vi "pmu_Build Class CFG.vi"(8 "error in (no error)":errorcluster, 11 "CFG input":T1={"PMU ID"=0, "time base"=10000000, "nominal frequency"=enum."60 Hz", "reporting rate"=60, "station name"="", "data format"=15, "phasor channels"=[], "analog channels"=[], "digital channels"=[]} {"digital channels"."digital unit" format="%08x"; "analog channels"."analog unit" format="%08x"; "phasor channels"."phasor unit scaling" max=16777215 format="%06x"; "phasor channels"."phasor unit" items=["Voltage [V]"=0, "Current [A]"=16777216]; "data format" format="%016b"}) -> (0 "error out":errorcluster, 3 "CFG class":T5={"station name"="", "PMU ID"=0, "time base"=10000000, "nominal frequency"=enum."60 Hz", "reporting rate"=60, "phasor number"=0, "analog number"=0, "digital number"=0, "channel names"=[], "phasor units"=[], "analog units"=[], "digital units"=[], "data format"=15, "number of PMUs"=1} {"digital units" format="%.0x"; "analog units" format="%.0x"; "phasor units" format="%.0x"})   [LabVIEW 2013, in "NI_EP_PMU.lvlib"]
uses:
  <vilib>/addons/Electrical Power/PMU/NI_EP_PMU.lvlib
  <vilib>/addons/Electrical Power/PMU/Common/Controls/pmu_CFG Class.ctl
  <vilib>/addons/Electrical Power/PMU/Common/Controls/pmu_CFG Input.ctl
  <vilib>/addons/Electrical Power/PMU/Common/Controls/pmu_Phasor Channel.ctl
  <vilib>/addons/Electrical Power/PMU/Common/Controls/pmu_Analog Channel.ctl
  <vilib>/addons/Electrical Power/PMU/Common/Controls/pmu_Digital Channel.ctl
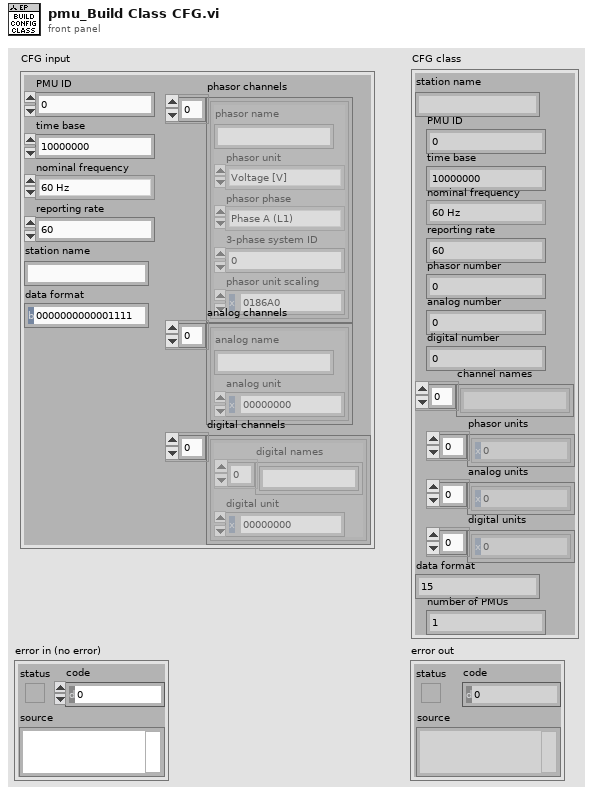
[diagram p1: front panel]
types:
  T1 = typedef "NI_EP_PMU.lvlib/pmu_CFG Input.ctl" = cluster{"PMU ID":u16, "time base":u32, "nominal frequency":enum16{"50 Hz", "60 Hz"}, "reporting rate":i16, "station name":string, "data format":u16, "phasor channels":T2[], "analog channels":T3[], "digital channels":T4[]}
  T2 = typedef "NI_EP_PMU.lvlib/pmu_Phasor Channel.ctl" = cluster{"phasor name":string, "phasor unit":u32, "phasor phase":enum16{"Phase A (L1)", "Phase B (L2)", "Phase C (L3)", "Phase N", "Positive sequence", "Negative sequence", "Zero sequence"}, "3-phase system ID":u8, "phasor unit scaling":u32}
  T3 = typedef "NI_EP_PMU.lvlib/pmu_Analog Channel.ctl" = cluster{"analog name":string, "analog unit":u32}
  T4 = typedef "NI_EP_PMU.lvlib/pmu_Digital Channel.ctl" = cluster{"digital names":string[], "digital unit":u32}
  T5 = typedef "NI_EP_PMU.lvlib/pmu_CFG Class.ctl" = cluster{"station name":string, "PMU ID":u16, "time base":u32, "nominal frequency":enum16{"50 Hz", "60 Hz"}, "reporting rate":i16, "phasor number":u16, "analog number":u16, "digital number":u16, "channel names":string[], "phasor units":u32[], "analog units":u32[], "digital units":u32[], "data format":u16, "number of PMUs":u16}
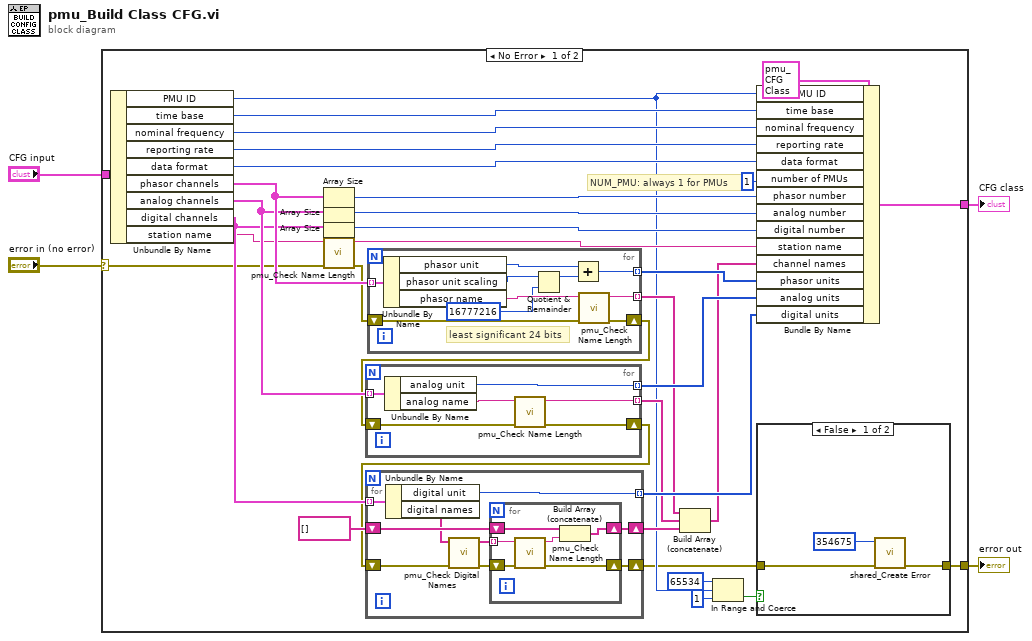
[diagram p0: block diagram]
diagram:
  n1 = case shown="No Error" "error in (no error)" {
    selector: "error in (no error)" -> [w12 w74]
    tunnel: "CFG input" -> [w37 _]
    tunnel: [w32 _] -> w3
    tunnel: [w7 w74] -> w1
    frame No Error {
      # "NUM_PMU: always 1 for PMUs"
      n2 = Unbundle By Name(w37) -> ("PMU ID"=w9:u16, "time base"=w36:u32, "nominal frequency"=w35:enum16{"50 Hz", "60 Hz"}, "reporting rate"=w34:i16, "data format"=w33:u16, "phasor channels"=w25:T2[], "analog channels"=w24:T3[], "digital channels"=w23:T4[], "station name"=w19:string)
      n3 = Array Size(array=w25) -> (size(s)=w22:i32)
      n4 = Array Size(array=w24) -> (size(s)=w21:i32)
      n5 = Array Size(array=w23) -> (size(s)=w20:i32)
      n6 = call <vilib>:"pmu_Check Name Length.vi"("error in (no error)"=w12, "name in"=w19) -> ("error out"=w17:errorcluster, "name out"=w18:string)  [unwired: 8 in]
      n7 = for {
        tunnel: w25 -> [w73] mode=indexing
        tunnel: [w71] -> w31 mode=indexing
        shift-right: [w69] -> w16
        shift-left: w17 -> [w70]
        tunnel: [w64] -> w14 mode=indexing
        # "least significant 24 bits"
        n8 = Unbundle By Name(w73) -> ("phasor unit"=w72:u32, "phasor unit scaling"=w67:u32, "phasor name"=w68:string)
        n9 = Quotient & Remainder(x=w67, y=u32 16777216) -> (x-y*floor(x/y)=w66:u32)  [unwired: 1 out]
        n10 = Add(x=w72, y=w66) -> (x+y=w71:u32)
        n11 = call <vilib>:"pmu_Check Name Length.vi"("error in (no error)"=w70, "name in"=w68) -> ("error out"=w69:errorcluster, "name out"=w64:string)  [unwired: 8 in]
      }
      n12 = for {
        tunnel: w24 -> [w63] mode=indexing
        tunnel: [w62] -> w30 mode=indexing
        shift-right: [w61] -> w15
        shift-left: w16 -> [w60]
        tunnel: [w58] -> w13 mode=indexing
        n13 = Unbundle By Name(w63) -> ("analog unit"=w62:u32, "analog name"=w59:string)
        n14 = call <vilib>:"pmu_Check Name Length.vi"("error in (no error)"=w60, "name in"=w59) -> ("error out"=w61:errorcluster, "name out"=w58:string)  [unwired: 8 in]
      }
      n15 = for {
        tunnel: w23 -> [w51] mode=indexing
        tunnel: [w50] -> w29 mode=indexing
        shift-right: [w47] -> w27
        shift-left: string[] [] ("element") -> [w48]
        shift-right: [w49] -> w6
        shift-left: w15 -> [w43]
        n16 = Unbundle By Name(w51) -> ("digital unit"=w50:u32, "digital names"=w46:string[])
        n17 = call <vilib>:"pmu_Check Digital Names.vi"("error in (no error)"=w43, "digital names in"=w46) -> ("error out"=w44:errorcluster, "digital names out"=w45:string[])  [unwired: 8 in]
        n18 = for {
          tunnel: w45 -> [w57] mode=indexing
          shift-right: [w55] -> w49
          shift-left: w44 -> [w56]
          shift-right: [w52] -> w47
          shift-left: w48 -> [w53]
          n19 = call <vilib>:"pmu_Check Name Length.vi"("error in (no error)"=w56, "name in"=w57) -> ("error out"=w55:errorcluster, "name out"=w54:string)  [unwired: 8 in]
          n20 = Build Array (concatenate)(w53, w54) -> (w52:string[])
        }
      }
      n21 = Build Array (concatenate)(w14, w13, w27) -> (w26:string[])
      n22 = In Range and Coerce(upper limit=u16 65534, x=w9, lower limit=u16 1) -> (In Range?=w8:bool)  [unwired: 1 out]
      n23 = Bundle By Name(cluster=T5 {"station name"="", "PMU ID"=0, "time base"=0, "nominal frequency"=enum."50 Hz", "reporting rate"=0, "phasor number"=0, "analog number"=0, "digital number"=0, "channel names"=[], "phasor units"=[], "analog units"=[], "digital units"=[], "data format"=0, "number of PMUs"=0} ("CFG class"), "PMU ID"=w9, "time base"=w36, "nominal frequency"=w35, "reporting rate"=w34, "data format"=w33, "number of PMUs"=u16 1, "phasor number"=w22, "analog number"=w21, "digital number"=w20, "station name"=w18, "channel names"=w26, "phasor units"=w31, "analog units"=w30, "digital units"=w29) -> (w32:T5)
      n24 = case shown="False" w8 {
        tunnel: [w39 w42] -> w7
        tunnel: w6 -> [w40 w42]
        frame False {
          n25 = call <vilib>:"shared_Create Error.vi"("error in (no error)"=w40, "error code (0)"=354675 ("code")) -> ("error out"=w39:errorcluster)  [unwired: 9 in]
        }
        frame True {
        }
      }
    }
    frame Error {
    }
  }
  "CFG class" <- w3
  "error out" <- w1
